vi "ParseSpec.vi"(8 "error in (no error)":errorcluster, 11 "Spec XML":string="<?xml version=\"1.0\" encoding=\"utf-8\"?>\n<Medulla>\n  <Doctype>Result</Doctype>\n  <Checksum>8765544332</Checksum>\n  <DriverKey>86y2e783he87</DriverKey>\n  <SpecId>1234567</SpecId>\n  <TransactionId>672362836</TransactionId>\n  <AccountID>Audinate</AccountID>\n  <SpecName>QF_TestSpec_CI24RE</SpecName>\n  <WorkflowStep>Test_CoilQF</WorkflowStep>\n  <SerialNumber>87362736</SerialNumber>\n  <BatchNumber>ase</BatchNumber>\n  <Status>Pass</Status>\n  <Comment>Repaired Unit</Comment>\n  <FirstFail>42344</FirstFail>\n  <Employee>Kurt</Employee>\n  <LocalMachine>QTS_Rig_1</LocalMachine>\n  <ResourceKey>12yu2yheiuh3</ResourceKey>\n  <Date>18/7/17</Date>\n  <Time>13:23:56</Time>\n  <Duration>00:1:27</Duration>\n  <DUTPosition>1</DUTPosition>\n  <Components>\n    <Component>\n      <SerialNumber>23214</SerialNumber>\n      <PartNumber>1234</PartNumber>\n      <Revision>A</Revision>\n      <BatchNumber></BatchNumber>\n      <Name>Grism</Name>\n      <Description>The Grism</Description>\n      <Attached>No</Attached>\n    </Component>\n    <Component>\n      <SerialNumber>464646646</SerialNumber>\n      <PartNumber>3456</PartNumber>\n      <Revision>B</Revision>\n      <BatchNumber></BatchNumber>\n      <Name>Prism</Name>\n      <Description>The Prism</Description>\n      <Attached>Yes</Attached>\n    </Component>\n  </Components>\n  <Attributes>\n    <Attribute>\n      <Name>Address</Name>\n      <Description>The IP of the Unit</Description>\n      <DataType>String</DataType>\n      <Value>192.168.1.7</Value>\n<DisplayFormat>%.3f</DisplayFormat>\n      <Access>R</Access>\n      <Required>NA</Required>\n    </Attribute>\n    <Attribute>\n      <Name>BaudRate</Name>\n      <Description>Baud rate of com port</Description>\n      <DataType>Int</DataType>\n      <Value>9600</Value>\n<DisplayFormat></DisplayFormat>\n      <Access>W</Access>\n      <Required>Yes</Required>\n    </Attribute>\n    <Attribute>\n      <Name>Switch State</Name>\n      <Description>State of the switch</Description>\n      <DataType>Boolean</DataType>\n      <Value>True</Value>\n<DisplayFormat></DisplayFormat>\n      <Access>W</Access>\n      <Required>No</Required>\n    </Attribute>\n  </Attributes>\n  <Tests>\n    <Test>\n      <Code>1</Code>\n      <Name>QFM Tests</Name>\n      <Description>blah</Description>\n      <Group></Group>\n      <IsGroup>Yes</IsGroup>\n      <Tag>QFM Tests</Tag>\n      <Method></Method>\n      <Parameter />\n      <DataType>Boolean</DataType>\n      <Value>1</Value>\n      <Status>Pass</Status>\n      <LimitLo></LimitLo>\n      <LimitHi></LimitHi>\n      <StringMatch></StringMatch>\n      <BooleanMatch>1</BooleanMatch>\n      <DisplayFormat></DisplayFormat>\n      <Units></Units>\n      <TestTime>00:01:27</TestTime>\n    </Test>\n    <Test>\n      <Code>1.1</Code>\n      <Name>Test Signal Strength</Name>\n      <Description>Test the signal strength</Description>\n      <Group>QFM Tests</Group>\n      <IsGroup>No</IsGroup>\n      <Tag>QFM Tests:Test Signal Strength</Tag>\n      <Method>Test_Sig</Method>\n      <Parameter />\n      <DataType>Int</DataType>\n      <Value>34.56</Value>\n      <Status>Pass</Status>\n      <LimitLo>25</LimitLo>\n      <LimitHi>100</LimitHi>\n      <StringMatch></StringMatch>\n      <BooleanMatch></BooleanMatch>\n      <DisplayFormat>%d</DisplayFormat>\n      <Units>Watts</Units>\n      <TestTime>00:00:45</TestTime>\n    </Test>\n    <Test>\n      <Code>1.2</Code>\n      <Name>Test Signal Frequency</Name>\n      <Description>Test the signal frequency</Description>\n      <Group>QFM Tests</Group>\n      <IsGroup>No</IsGroup>\n      <Tag>QFM Tests:Test Signal Frequency</Tag>\n      <Method>Test_Freq</Method>\n      <Parameter />\n      <DataType>Dbl</DataType>\n      <Value>45.67</Value>\n      <Status>Pass</Status>\n      <LimitLo>45</LimitLo>\n      <LimitHi>46</LimitHi>\n      <StringMatch></StringMatch>\n      <BooleanMatch></BooleanMatch>\n      <DisplayFormat>%.3f</DisplayFormat>\n      <Units>MHz</Units>\n      <TestTime>00:00:20</TestTime>\n    </Test>\n    <Test>\n      <Code>Code</Code>\n      <Name>Test Firmware Vesion</Name>\n      <Description>Test the Firmware Vesion</Description>\n      <Group>QFM Tests</Group>\n      <IsGroup>No</IsGroup>\n      <Tag>QFM Tests:Test Firmware Vesion</Tag>\n      <Method>Test_FWVer</Method>\n      <Parameter />\n      <DataType>String</DataType>\n      <Value>Ver1.2</Value>\n      <Status>Pass</Status>\n      <LimitLo></LimitLo>\n      <LimitHi></LimitHi>\n      <StringMatch>Ver1.2</StringMatch>\n      <BooleanMatch></BooleanMatch>\n      <DisplayFormat></DisplayFormat>\n      <Units></Units>\n      <TestTime>00:00:12</TestTime>\n    </Test>\n    <Test>\n      <Code>Test LED State</Code>\n      <Name>Test LED State</Name>\n      <Description>Tests that the LED is On</Description>\n      <Group>QFM Tests</Group>\n      <IsGroup>No</IsGroup>\n      <Tag>QFM Tests:Test LED State</Tag>\n      <Method>Test_LED</Method>\n      <Parameter />\n      <DataType>Boolean</DataType>\n      <Value>True</Value>\n      <Status>Pass</Status>\n      <LimitLo></LimitLo>\n      <LimitHi></LimitHi>\n      <StringMatch></StringMatch>\n      <BooleanMatch>True</BooleanMatch>\n      <DisplayFormat></DisplayFormat>\n      <Units></Units>\n      <TestTime>00:00:10</TestTime>\n    </Test>\n  </Tests>\n</Medulla>") -> (0 "error out":errorcluster, 3 "Spec":T1)   [LabVIEW 2022 SP3, in "MES_Base.lvlib" / "MES_Base.lvclass"]
uses:
  MES_Base.lvclass
  Controls/Spec.ctl
  Controls/SpecHeader.ctl
  Controls/Status.ctl
  Controls/SpecComponent.ctl
  Controls/SpecAttribute.ctl
  Controls/DataType.ctl
  Controls/Test.ctl
  <vilib>/xml/Load XML String.vi
  <vilib>/xml/Close Reference(Node).vi
  <vilib>/xml/NI_XML.lvlib
panel:
  # "<SerialNumber>23214</SerialNumber>\n      <PartNumber>1234</PartNumber>\n      <Revision>A</Revision>\n      <BatchNumber></BatchNumber>\n      <Name>Grism</Name>\n      <Description>The Grism</Description>\n      <Attached>Yes</Attached>"
  # "<Attribute>\n      <Name>Address</Name>\n      <Description>The IP of the Unit</Description>\n      <DataType>String</DataType>\n      <Value>192.168.1.7</Value>\n      <Access>R</Access>\n      <Required>NA</Required>\n    </Attribute>"
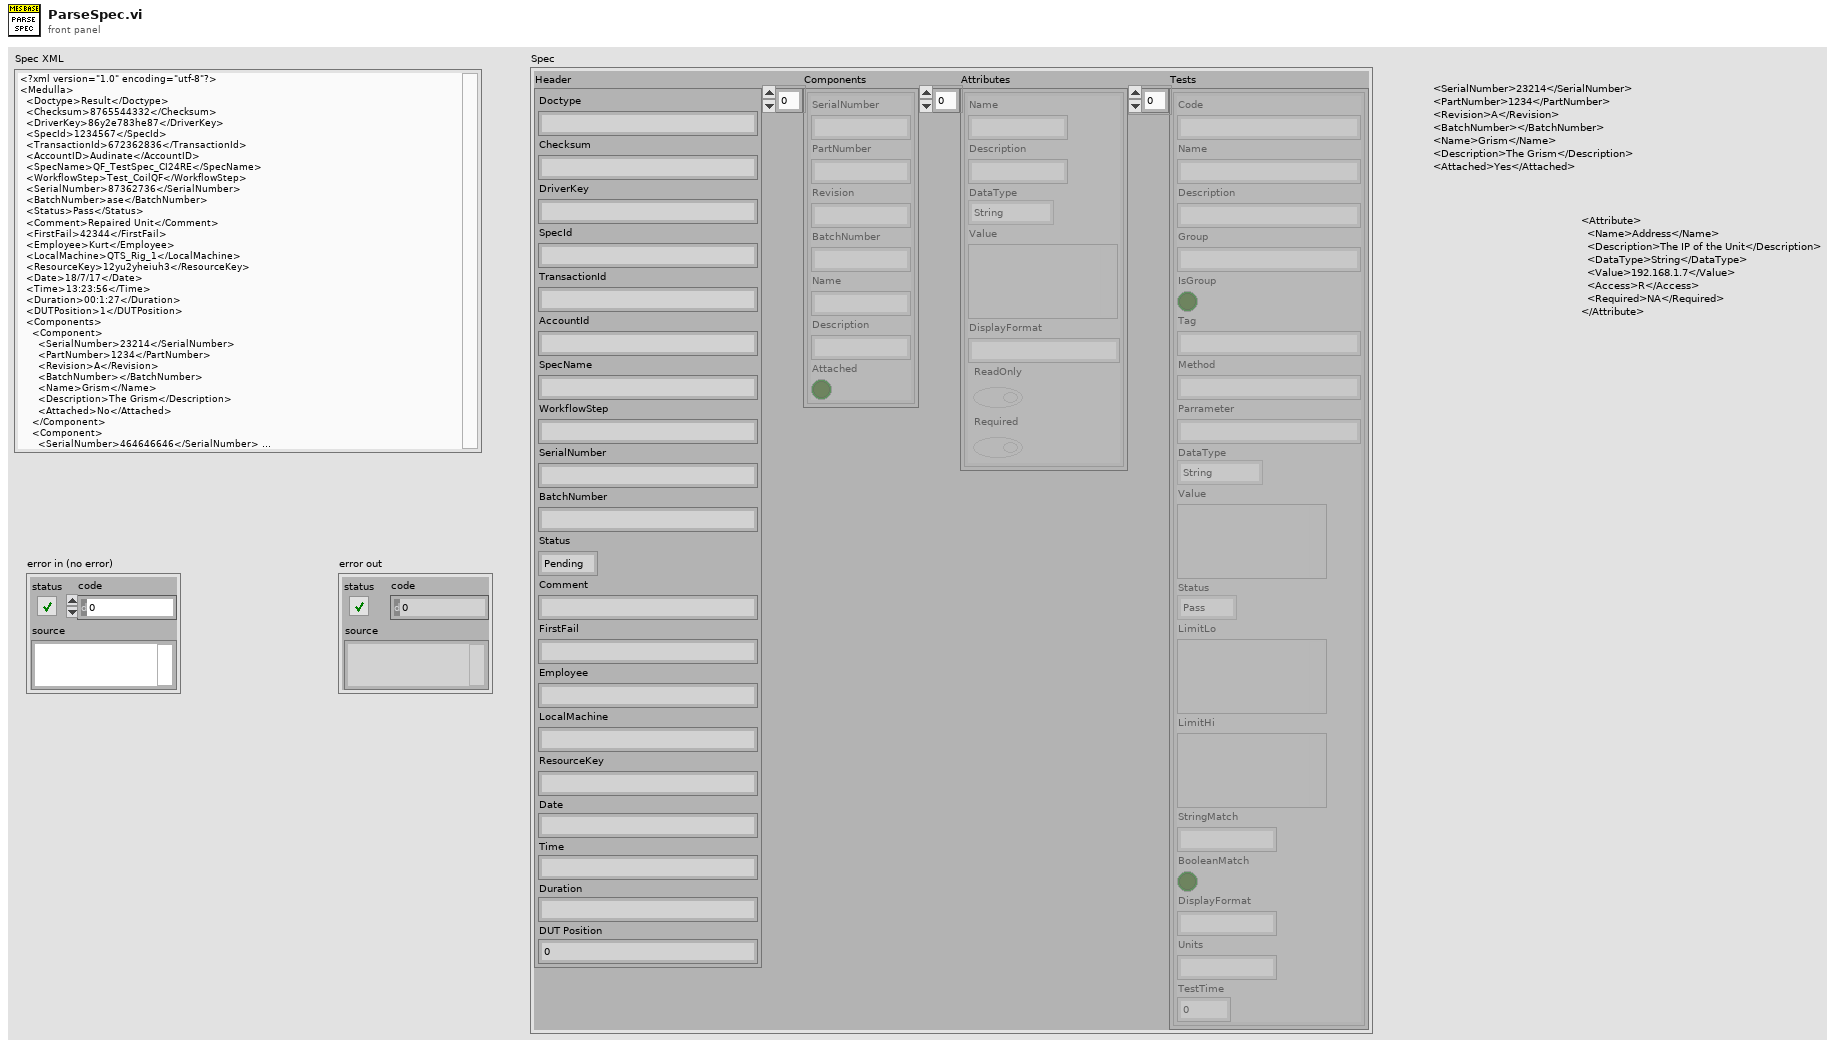
[diagram p1: front panel]
types:
  T1 = typedef "MES_Base.lvlib/MES_Base.lvclass/Spec.ctl" = cluster{"Header":T2, "Components":T4[], "Attributes":T5[], "Tests":T7[]}
  T2 = typedef "MES_Base.lvlib/MES_Base.lvclass/SpecHeader.ctl" = cluster{"Doctype":string, "Checksum":string, "DriverKey":string, "SpecId":string, "TransactionId":string, "AccountId":string, "SpecName":string, "WorkflowStep":string, "SerialNumber":string, "BatchNumber":string, "Status":T3, "Comment":string, "FirstFail":string, "Employee":string, "LocalMachine":string, "ResourceKey":string, "Date":string, "Time":string, "Duration":string, "DUT Position":i32}
  T3 = typedef "MES_Base.lvlib/MES_Base.lvclass/Status.ctl" = enum16{"Pending", "Pass", "Fail"}
  T4 = typedef "MES_Base.lvlib/MES_Base.lvclass/SpecComponent.ctl" = cluster{"SerialNumber":string, "PartNumber":string, "Revision":string, "BatchNumber":string, "Name":string, "Description":string, "Attached":bool}
  T5 = typedef "MES_Base.lvlib/MES_Base.lvclass/SpecAttribute.ctl" = cluster{"Name":string, "Description":string, "DataType":T6, "Value":variant, "DisplayFormat":string, "ReadOnly":bool, "Required":bool}
  T6 = typedef "MES_Base.lvlib/MES_Base.lvclass/DataType.ctl" = enum16{"NA", "String", "Boolean", "Int", "Dbl"}
  T7 = typedef "MES_Base.lvlib/MES_Base.lvclass/Test.ctl" = cluster{"Code":string, "Name":string, "Description":string, "Group":string, "IsGroup":bool, "Tag":string, "Method":string, "Parrameter":string, "DataType":T6, "Value":variant, "Status":T3, "LimitLo":variant, "LimitHi":variant, "StringMatch":string, "BooleanMatch":bool, "DisplayFormat":string, "Units":string, "TestTime":dbl}
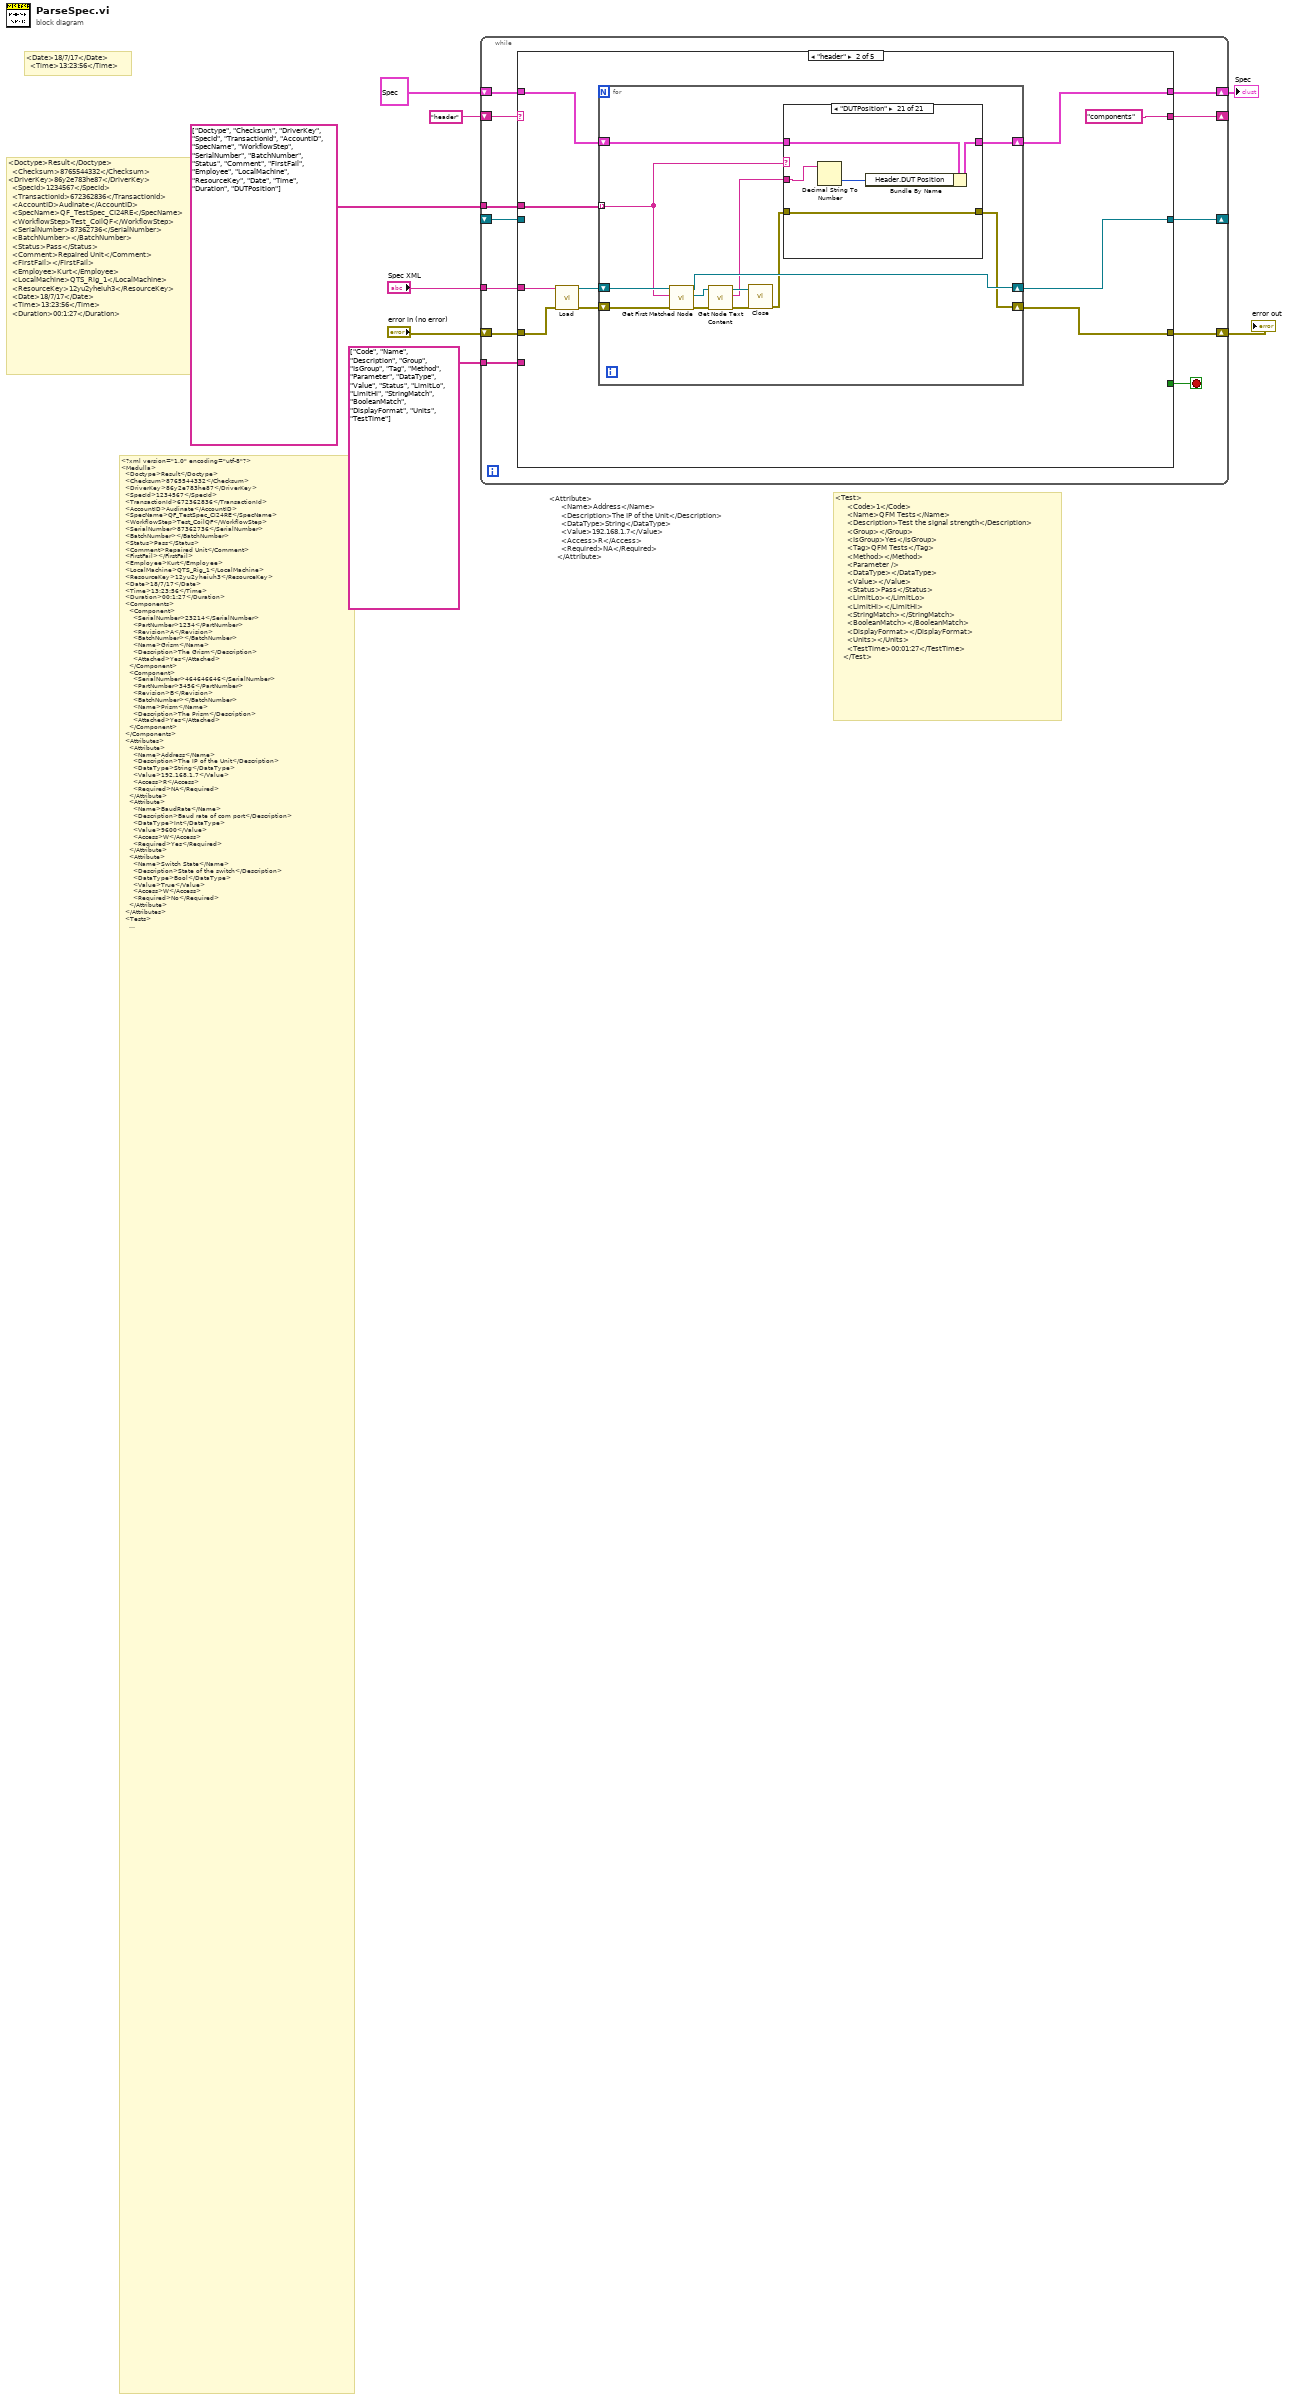
[diagram p0: block diagram]
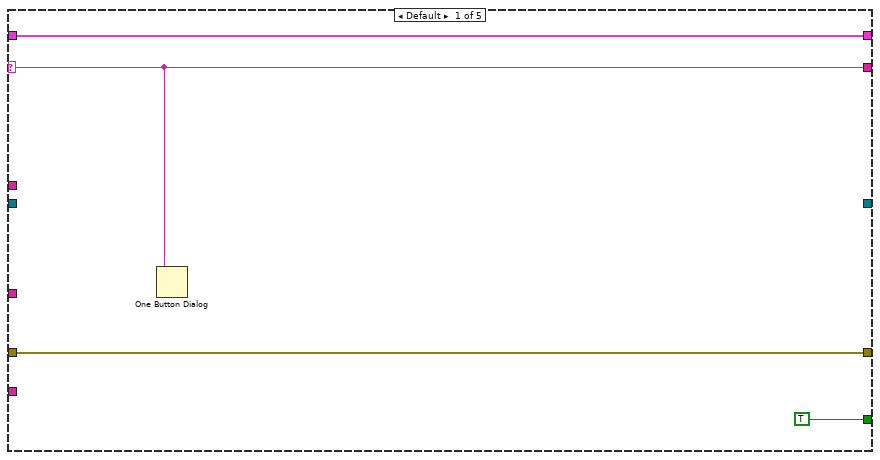
[diagram p2: hidden frame]
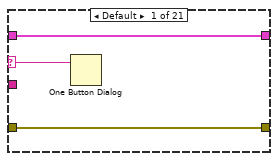
[diagram p3: hidden frame]
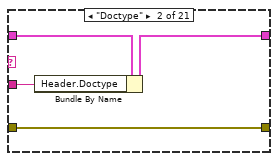
[diagram p4: hidden frame]
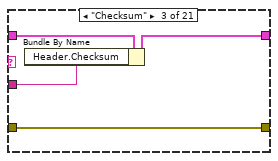
[diagram p5: hidden frame]
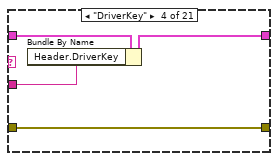
[diagram p6: hidden frame]
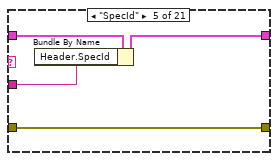
[diagram p7: hidden frame]
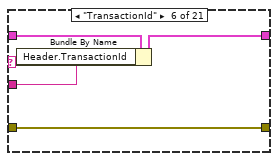
[diagram p8: hidden frame]
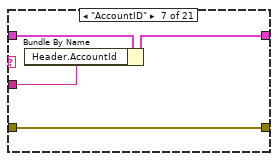
[diagram p9: hidden frame]
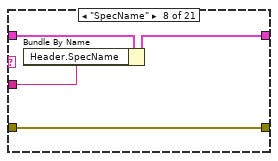
[diagram p10: hidden frame]
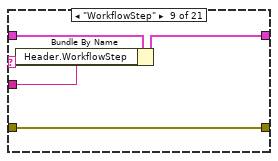
[diagram p11: hidden frame]
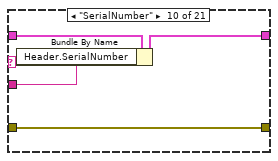
[diagram p12: hidden frame]
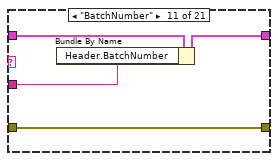
[diagram p13: hidden frame]
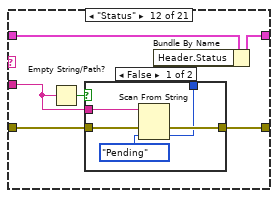
[diagram p14: hidden frame]
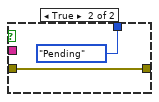
[diagram p15: hidden frame]
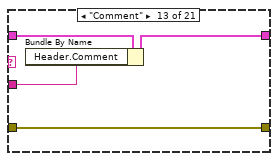
[diagram p16: hidden frame]
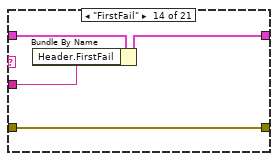
[diagram p17: hidden frame]
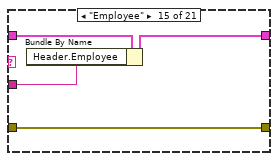
[diagram p18: hidden frame]
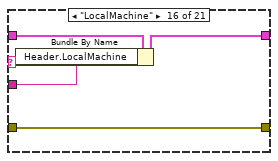
[diagram p19: hidden frame]
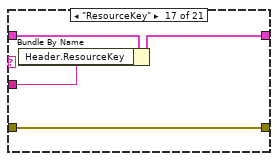
[diagram p20: hidden frame]
diagram:
  # "<Date>18/7/17</Date>\n  <Time>13:23:56</Time>"
  # "<Test>\n      <Code>1</Code>\n      <Name>QFM Tests</Name>\n      <Description>Test the signal strength</Description>\n      <Group></Group>\n      <IsGroup>Yes</IsGroup>\n      <Tag>QFM Tests</Tag>\n      <Method></Method>\n      <Parameter />\n      <DataType></DataType>\n      <Value></Value>\n      <Status>Pass</Status>\n      <LimitLo></LimitLo>\n      <LimitHi></LimitHi>\n      <StringMatch></StringMatch>\n      <BooleanMatch></BooleanMatch>\n      <DisplayFormat></DisplayFormat>\n      <Units></Units>\n      <TestTime>00:01:27</TestTime>\n    </Test>"
  # "<Attribute>\n      <Name>Address</Name>\n      <Description>The IP of the Unit</Description>\n      <DataType>String</DataType>\n      <Value>192.168.1.7</Value>\n      <Access>R</Access>\n      <Required>NA</Required>\n    </Attribute>"
  # "<Doctype>Result</Doctype>\n  <Checksum>8765544332</Checksum>\n<DriverKey>86y2e783he87</DriverKey>\n  <SpecId>1234567</SpecId>\n  <TransactionId>672362836</TransactionId>\n  <AccountID>Audinate</AccountID>\n  <SpecName>QF_TestSpec_CI24RE</SpecName>\n  <WorkflowStep>Test_CoilQF</WorkflowStep>\n  <SerialNumber>87362736</SerialNumber>\n  <BatchNumber></BatchNumber>\n  <Status>Pass</Status>\n  <Comment>Repaired Unit</Comment>\n  <FirstFail></FirstFail>\n  <Employee>Kurt</Employee>\n  <LocalMachine>QTS_Rig_1</LocalMachine>\n  <ResourceKey>12yu2yheiuh3</ResourceKey>\n  <Date>18/7/17</Date>\n  <Time>13:23:56</Time>\n  <Duration>00:1:27</Duration>"
  # "<?xml version=\"1.0\" encoding=\"utf-8\"?>\n<Medulla>\n  <Doctype>Result</Doctype>\n  <Checksum>8765544332</Checksum>\n  <DriverKey>86y2e783he87</DriverKey>\n  <SpecId>1234567</SpecId>\n  <TransactionId>672362836</TransactionId>\n  <AccountID>Audinate</AccountID>\n  <SpecName>QF_TestSpec_CI24RE</SpecName>\n  <WorkflowStep>Test_CoilQF</WorkflowStep>\n  <SerialNumber>87362736</SerialNumber>\n  <BatchNumber></BatchNumber>\n  <Status>Pass</Status>\n  <Comment>Repaired Unit</Comment>\n  <FirstFail></FirstFail>\n  <Employee>Kurt</Employee>\n  <LocalMachine>QTS_Rig_1</LocalMachine>\n  <ResourceKey>12yu2yheiuh3</ResourceKey>\n  <Date>18/7/17</Date>\n  <Time>13:23:56</Time>\n  <Duration>00:1:27</Duration>\n  <Components>\n    <Component>\n      <SerialNumber>23214</SerialNumber>\n      <PartNumber>1234</PartNumber>\n      <Revision>A</Revision>\n      <BatchNumber></BatchNumber>\n      <Name>Grism</Name>\n      <Description>The Grism</Description>\n      <Attached>Yes</Attached>\n    </Component>\n    <Component>\n      <SerialNumber>464646646</SerialNumber>\n      <PartNumber>3456</PartNumber>\n      <Revision>B</Revision>\n      <BatchNumber></BatchNumber>\n      <Name>Prism</Name>\n      <Description>The Prism</Description>\n      <Attached>Yes</Attached>\n    </Component>\n  </Components>\n  <Attributes>\n    <Attribute>\n      <Name>Address</Name>\n      <Description>The IP of the Unit</Description>\n      <DataType>String</DataType>\n      <Value>192.168.1.7</Value>\n      <Access>R</Access>\n      <Required>NA</Required>\n    </Attribute>\n    <Attribute>\n      <Name>BaudRate</Name>\n      <Description>Baud rate of com port</Description>\n      <DataType>Int</DataType>\n      <Value>9600</Value>\n      <Access>W</Access>\n      <Required>Yes</Required>\n    </Attribute>\n    <Attribute>\n      <Name>Switch State</Name>\n      <Description>State of the switch</Description>\n      <DataType>Bool</DataType>\n      <Value>True</Value>\n      <Access>W</Access>\n      <Required>No</Required>\n    </Attribute>\n  </Attributes>\n  <Tests>\n    <Test>\n      <Code>1</Code>\n      <Name>QFM Tests</Name>\n      <Description>Test the signal strength</Description>\n      <Group></Group>\n      <IsGroup>Yes</IsGroup>\n      <Tag>QFM Tests</Tag>\n      <Method></Method>\n      <Parameter />\n      <DataType></DataType>\n      <Value></Value>\n      <Status>Pass</Status>\n      <LimitLo></LimitLo>\n      <LimitHi></LimitHi>\n      <StringMatch></StringMatch>\n      <BooleanMatch></BooleanMatch>\n      <DisplayFormat></DisplayFormat>\n      <Units></Units>\n      <TestTime>00:01:27</TestTime>\n    </Test>\n    <Test>\n      <Code>1.1</Code>\n      <Name>Test Signal Strength</Name>\n      <Description>Test the signal strength</Description>\n      <Group>QFM Tests</Group>\n      <IsGroup>No</IsGroup>\n      <Tag>QFM Tests:Test Signal Strength</Tag>\n      <Method>Test_Sig</Method>\n      <Parameter />\n      <DataType>Int</DataType>\n      <Value>34.56</Value>\n      <Status>Pass</Status>\n      <LimitLo>25</LimitLo>\n      <LimitHi>100</LimitHi>\n      <StringMatch></StringMatch>\n      <BooleanMatch></BooleanMatch>\n      <DisplayFormat>%d</DisplayFormat>\n      <Units>Watts</Units>\n      <TestTime>00:00:45</TestTime>\n    </Test>\n    <Test>\n      <Code>1.2</Code>\n      <Name>Test Signal Frequency</Name>\n      <Description>Test the signal frequency</Description>\n      <Group>QFM Tests</Group>\n      <IsGroup>No</IsGroup>\n      <Tag>QFM Tests:Test Signal Frequency</Tag>\n      <Method>Test_Freq</Method>\n      <Parameter />\n      <DataType>DBL</DataType>\n      <Value>45.67</Value>\n      <Status>Pass</Status>\n      <LimitLo>45</LimitLo>\n      <LimitHi>46</LimitHi>\n      <StringMatch></StringMatch>\n      <BooleanMatch></BooleanMatch>\n      <DisplayFormat>%.3f</DisplayFormat>\n      <Units>MHz</Units>\n      <TestTime>00:00:20</TestTime>\n    </Test>\n    <Test>\n      <Code>Code</Code>\n      <Name>Test Firmware Vesion</Name>\n      <Description>Test the Firmware Vesion</Description>\n      <Group>QFM Tests</Group>\n      <IsGroup>No</IsGroup>\n      <Tag>QFM Tests:Test Firmware Vesion</Tag>\n      <Method>Test_FWVer</Method>\n      <Parameter />\n      <DataType>String</DataType>\n      <Value>Ver1.2</Value>\n      <Status>Pass</Status>\n      <LimitLo></LimitLo>\n      <LimitHi></LimitHi>\n      <StringMatch>Ver1.2</StringMatch>\n      <BooleanMatch></BooleanMatch>\n      <DisplayFormat></DisplayFormat>\n      <Units></Units>\n      <TestTime>00:00:12</TestTime>\n    </Test>\n    <Test>\n      <Code>Test LED State</Code>\n      <Name>Test LED State</Name>\n      <Description>Tests that the LED is On</Description>\n      <Group>QFM Tests</Group>\n      <IsGroup>No</IsGroup>\n      <Tag>QFM Tests:Test LED State</Tag>\n      <Method>Test_LED</Method>\n      <Parameter />\n      <DataType>Boolean</DataType>\n      <Value>True</Value>\n      <Status>True</Status>\n      <LimitLo></LimitLo>\n      <LimitHi></LimitHi>\n      <StringMatch></StringMatch>\n      <BooleanMatch>True</BooleanMatch>\n      <DisplayFormat></DisplayFormat>\n      <Units></Units>\n      <TestTime>00:00:10</TestTime>\n    </Test>\n  </Tests>\n</Medulla>"
  n1 = while {
    shift-right: [w15] -> w4
    shift-left: "error in (no error)" -> [w19]
    tunnel: "Spec XML" -> [w18]
    shift-right: [w13] -> _
    shift-left: "header" -> [w20]
    shift-right: [w14] -> w2
    shift-left: T1 {"Header"={"Doctype"="", "Checksum"="", "DriverKey"="", "SpecId"="", "TransactionId"="", "AccountId"="", "SpecName"="", "WorkflowStep"="", "SerialNumber"="", "BatchNumber"="", "Status"=enum."Pending", "Comment"="", "FirstFail"="", "Employee"="", "LocalMachine"="", "ResourceKey"="", "Date"="", "Time"="", "Duration"="", "DUT Position"=0}, "Components"=[], "Attributes"=[], "Tests"=[]} ("Spec") -> [w17]
    tunnel: string[] ["Doctype", "Checksum", "DriverKey", "SpecId", "TransactionId", "AccountID", "SpecName", "WorkflowStep", "SerialNumber", "BatchNumber", "Status", "Comment", "FirstFail", "Employee", "LocalMachine", "ResourceKey", "Date", "Time", "Duration", "DUTPosition"] -> [w16]
    shift-right: [w11] -> _
    shift-left: _ -> [w10]
    tunnel: string[] ["Code", "Name", "Description", "Group", "IsGroup", "Tag", "Method", "Parameter", "DataType", "Value", "Status", "LimitLo", "LimitHi", "StringMatch", "BooleanMatch", "DisplayFormat", "Units", "TestTime"] -> [w9]
    stop <- w12 stop-if-true
    n2 = case shown="\"header\"" w20 {
      selector: w20 -> [w21 _ _ _ _]
      tunnel: w19 -> [w24 w33 w152 w204 w286]
      tunnel: w18 -> [_ w34 _ _ _]
      tunnel: w17 -> [w22 w29 w146 w198 w281]
      tunnel: w16 -> [_ w30 _ _ _]
      tunnel: [w24 w28 w148 w200 w282] -> w15
      tunnel: [w22 w27 w145 w197 w280] -> w14
      tunnel: [w21 "components" "attributes" "tests" "done"] -> w13
      tunnel: [TRUE _ _ _ TRUE] -> w12
      tunnel: [_ w25 w143 w195 w278] -> w11
      tunnel: w10 -> [_ _ w143 w195 w278]
      tunnel: w9 -> [_ _ _ _ w276]
      frame Default {
        n3 = One Button Dialog(message=w21) -> ()  [unwired: 1 in, 1 out]
      }
      frame "header" {
        n4 = call-poly <vilib>:"Load.vi"("XML string"=w34, "error in (no error)"=w33) -> ("DOM document out"=w32:refnum<k20>, "error out"=w31:errorcluster)  [unwired: 11 in, 1 out]
        n5 = for {
          shift-right: [w35] -> w28
          shift-left: w31 -> [w38]
          tunnel: w30 -> [w37] mode=indexing
          shift-right: [w42] -> w25
          shift-left: w32 -> [w47]
          shift-right: [w39] -> w27
          shift-left: w29 -> [w41]
          n6 = call <vilib>:"Get First Matched Node.vi"("error in (no error)"=w38, "XPath expression"=w37, "node in"=w47) -> ("error out"=w46:errorcluster, "node result"=w45:refnum<k20>, "node out"=w42:refnum<k20>)  [unwired: 6 in]
          n7 = call <vilib>:"Get Node Text Content.vi"("error in (no error)"=w46, "node in"=w45) -> ("error out"=w44:errorcluster, "node text"=w40:string, "node out"=w43:refnum<k20>)  [unwired: 7 in]
          n8 = call-poly <vilib>:"Close.vi"("error in (no error)"=w44, "node"=w43) -> ("error out"=w36:errorcluster)  [unwired: 7 out]
          n9 = case shown="\"DUTPosition\"" w37 {
            selector: w37 -> [w49 _ _ _ _ _ _ _ _ _ _ _ _ _ _ _ _ _ _ _ _]
            tunnel: w41 -> [w50 w54 w58 w62 w66 w70 w74 w78 w82 w86 w90 w97 w108 w112 w116 w120 w124 w128 w132 w136 w141]
            tunnel: w40 -> [_ w52 w56 w60 w64 w68 w72 w76 w80 w84 w88 w93 w106 w110 w114 w118 w122 w126 w130 w134 w138]
            tunnel: [w50 w53 w57 w61 w65 w69 w73 w77 w81 w85 w89 w96 w107 w111 w115 w119 w123 w127 w131 w135 w140] -> w39
            tunnel: w36 -> [w48 w51 w55 w59 w63 w67 w71 w75 w79 w83 w87 w92 w105 w109 w113 w117 w121 w125 w129 w133 w139]
            tunnel: [w48 w51 w55 w59 w63 w67 w71 w75 w79 w83 w87 w91 w105 w109 w113 w117 w121 w125 w129 w133 w139] -> w35
            frame Default {
              n10 = One Button Dialog(message=w49) -> ()  [unwired: 1 in, 1 out]
            }
            frame "Doctype" {
              n11 = Bundle By Name(cluster=w54, "Header.Doctype"=w52) -> (w53:T1)
            }
            frame "Checksum" {
              n12 = Bundle By Name(cluster=w58, "Header.Checksum"=w56) -> (w57:T1)
            }
            frame "DriverKey" {
              n13 = Bundle By Name(cluster=w62, "Header.DriverKey"=w60) -> (w61:T1)
            }
            frame "SpecId" {
              n14 = Bundle By Name(cluster=w66, "Header.SpecId"=w64) -> (w65:T1)
            }
            frame "TransactionId" {
              n15 = Bundle By Name(cluster=w70, "Header.TransactionId"=w68) -> (w69:T1)
            }
            frame "AccountID" {
              n16 = Bundle By Name(cluster=w74, "Header.AccountId"=w72) -> (w73:T1)
            }
            frame "SpecName" {
              n17 = Bundle By Name(cluster=w78, "Header.SpecName"=w76) -> (w77:T1)
            }
            frame "WorkflowStep" {
              n18 = Bundle By Name(cluster=w82, "Header.WorkflowStep"=w80) -> (w81:T1)
            }
            frame "SerialNumber" {
              n19 = Bundle By Name(cluster=w86, "Header.SerialNumber"=w84) -> (w85:T1)
            }
            frame "BatchNumber" {
              n20 = Bundle By Name(cluster=w90, "Header.BatchNumber"=w88) -> (w89:T1)
            }
            frame "Status" {
              n21 = Empty String/Path?(string/path=w93) -> (empty?=w95:bool)
              n22 = case shown="False" w95 {
                tunnel: w92 -> [w102 w104]
                tunnel: [w101 w104] -> w91
                tunnel: [w99 Status."Pending" ("Status")] -> w94
                tunnel: w93 -> [w98 _]
                frame False {
                  n23 = Scan From String(input string=w98, error in=w102, default 1=Status."Pending" ("Status")) -> (error out=w101:errorcluster, output 1=w99:T3)  [unwired: 2 in, 2 out]
                }
                frame True {
                }
              }
              n24 = Bundle By Name(cluster=w97, "Header.Status"=w94) -> (w96:T1)
            }
            frame "Comment" {
              n25 = Bundle By Name(cluster=w108, "Header.Comment"=w106) -> (w107:T1)
            }
            frame "FirstFail" {
              n26 = Bundle By Name(cluster=w112, "Header.FirstFail"=w110) -> (w111:T1)
            }
            frame "Employee" {
              n27 = Bundle By Name(cluster=w116, "Header.Employee"=w114) -> (w115:T1)
            }
            frame "LocalMachine" {
              n28 = Bundle By Name(cluster=w120, "Header.LocalMachine"=w118) -> (w119:T1)
            }
            frame "ResourceKey" {
              n29 = Bundle By Name(cluster=w124, "Header.ResourceKey"=w122) -> (w123:T1)
            }
            frame "Date" {
              n30 = Bundle By Name(cluster=w128, "Header.Date"=w126) -> (w127:T1)
            }
            frame "Time" {
              n31 = Bundle By Name(cluster=w132, "Header.Time"=w130) -> (w131:T1)
            }
            frame "Duration" {
              n32 = Bundle By Name(cluster=w136, "Header.Duration"=w134) -> (w135:T1)
            }
            frame "DUTPosition" {
              n33 = Decimal String To Number(string=w138) -> (number=w137:i32)  [unwired: 2 in, 1 out]
              n34 = Bundle By Name(cluster=w141, "Header.DUT Position"=w137) -> (w140:T1)
            }
          }
        }
      }
      frame "components" {
        n35 = call <vilib>:"Get All Matched Nodes.vi"("error in (no error)"=w152, "XPath expression"="Components/Component", "node in"=w143) -> ("error out"=w150:errorcluster, "node result array"=w149:refnum<k20>[])  [unwired: 6 in, 1 out]
        n36 = for {
          shift-right: [w155] -> w148
          shift-left: w150 -> [w158]
          tunnel: w149 -> [w157] mode=indexing
          tunnel: string[] ["SerialNumber", "PartNumber", "Revision", "BatchNumber", "Name", "Description", "Attached"] -> [w156]
          tunnel: [w154] -> w144 mode=indexing
          n37 = for {
            tunnel: w157 -> [w168]
            tunnel: w156 -> [w162] mode=indexing
            shift-right: [w164] -> w155
            shift-left: w158 -> [w169]
            shift-right: [w160] -> w154
            shift-left: T4 {"SerialNumber"="", "PartNumber"="", "Revision"="", "BatchNumber"="", "Name"="", "Description"="", "Attached"=FALSE} ("Component") -> [w161]
            n38 = call <vilib>:"Get First Matched Node.vi"("error in (no error)"=w169, "XPath expression"=w162, "node in"=w168) -> ("error out"=w166:errorcluster, "node result"=w167:refnum<k20>)  [unwired: 6 in, 1 out]
            n39 = call <vilib>:"Get Node Text Content.vi"("error in (no error)"=w166, "node in"=w167) -> ("error out"=w165:errorcluster, "node text"=w159:string, "node out"=w163:refnum<k20>)  [unwired: 7 in]
            n40 = case shown="\"Revision\"" w162 {
              tunnel: w161 -> [w170 w173 w176 w179 w182 w185 w188 w193]
              tunnel: [w170 w172 w175 w178 w181 w184 w187 w192] -> w160
              tunnel: w159 -> [_ w171 w174 w177 w180 w183 w186 w191]
              frame Default {
              }
              frame "SerialNumber" {
                n41 = Bundle By Name(cluster=w173, "SerialNumber"=w171) -> (w172:T4)
              }
              frame "PartNumber" {
                n42 = Bundle By Name(cluster=w176, "PartNumber"=w174) -> (w175:T4)
              }
              frame "Revision" {
                n43 = Bundle By Name(cluster=w179, "Revision"=w177) -> (w178:T4)
              }
              frame "BatchNumber" {
                n44 = Bundle By Name(cluster=w182, "BatchNumber"=w180) -> (w181:T4)
              }
              frame "Name" {
                n45 = Bundle By Name(cluster=w185, "Name"=w183) -> (w184:T4)
              }
              frame "Description" {
                n46 = Bundle By Name(cluster=w188, "Description"=w186) -> (w187:T4)
              }
              frame "Attached" {
                n47 = Equal?(x="Yes", y=w191) -> (x = y?=w189:bool)
                n48 = Bundle By Name(cluster=w193, "Attached"=w189) -> (w192:T4)
              }
            }
            n49 = call-poly <vilib>:"Close.vi"("error in (no error)"=w165, "node"=w163) -> ("error out"=w164:errorcluster)  [unwired: 7 in]
          }
        }
        n50 = Bundle By Name(cluster=w146, "Components"=w144) -> (w145:T1)
      }
      frame "attributes" {
        n51 = call <vilib>:"Get All Matched Nodes.vi"("error in (no error)"=w204, "XPath expression"="Attributes/Attribute", "node in"=w195) -> ("error out"=w202:errorcluster, "node result array"=w201:refnum<k20>[])  [unwired: 6 in, 1 out]
        n52 = for {
          shift-right: [w207] -> w200
          shift-left: w202 -> [w210]
          tunnel: w201 -> [w209] mode=indexing
          tunnel: string[] ["Name", "Description", "DataType", "Value", "DisplayFormat", "Access", "Required"] -> [w208]
          tunnel: [w206] -> w196 mode=indexing
          n53 = for {
            tunnel: w209 -> [w221]
            tunnel: w208 -> [w216] mode=indexing
            shift-right: [w218] -> w207
            shift-left: w210 -> [w222]
            shift-right: [w214] -> w206
            shift-left: T5 {"Name"="", "Description"="", "DataType"=enum."String", "Value"=variant, "DisplayFormat"="", "ReadOnly"=FALSE, "Required"=FALSE} ("Attribute") -> [w215]
            n54 = call <vilib>:"Get First Matched Node.vi"("error in (no error)"=w222, "XPath expression"=w216, "node in"=w221) -> ("error out"=w219:errorcluster, "node result"=w220:refnum<k20>)  [unwired: 6 in, 1 out]
            n55 = call <vilib>:"Get Node Text Content.vi"("error in (no error)"=w219, "node in"=w220) -> ("error out"=w212:errorcluster, "node text"=w213:string, "node out"=w217:refnum<k20>)  [unwired: 7 in]
            n56 = case shown="\"DataType\"" w216 {
              tunnel: w215 -> [w224 w228 w232 w239 w243 w260 w268 w274]
              tunnel: [w224 w227 w231 w238 w245 w262 w267 w273] -> w214
              tunnel: w213 -> [_ w226 w230 w237 w241 w259 w266 w271]
              tunnel: w212 -> [w223 w225 w229 w235 w244 w261 w263 w269]
              tunnel: [w223 w225 w229 w234 w244 w261 w263 w269] -> w211
              frame Default {
              }
              frame "Name" {
                n57 = Bundle By Name(cluster=w228, "Name"=w226) -> (w227:T5)
              }
              frame "Description" {
                n58 = Bundle By Name(cluster=w232, "Description"=w230) -> (w231:T5)
              }
              frame "DataType" {
                n59 = Scan From String(input string=w237, error in=w235, default 1=DataType."Dbl" ("DataType")) -> (error out=w234:errorcluster, output 1=w236:T6)  [unwired: 2 in, 2 out]
                n60 = Bundle By Name(cluster=w239, "DataType"=w236) -> (w238:T5)
              }
              frame "Value" {
                n61 = Unbundle By Name(w243) -> ("DataType"=w242:T6)
                n62 = case shown="\"Dbl\"" w242 {
                  tunnel: w241 -> [w247 w251 w255 w257]
                  tunnel: [w246 w248 w252 w258] -> w240
                  frame "String", Default {
                    n63 = To Variant(anything=w247) -> (Variant=w246:variant)
                  }
                  frame "Boolean" {
                    n64 = Equal?(x="1", y=w251) -> (x = y?=w249:bool)
                    n65 = To Variant(anything=w249) -> (Variant=w248:variant)
                  }
                  frame "Int" {
                    n66 = Decimal String To Number(string=w255, default (0L)=i64 0 ("default (0 I32)")) -> (number=w253:i64)  [unwired: 1 in, 1 out]
                    n67 = To Variant(anything=w253) -> (Variant=w252:variant)
                  }
                  frame "Dbl" {
                    n68 = Fract/Exp String To Number(string=w257) -> (number=w256:dbl)  [unwired: 3 in, 1 out]
                    n69 = To Variant(anything=w256) -> (Variant=w258:variant)
                  }
                }
                n70 = Bundle By Name(cluster=w243, "Value"=w240) -> (w245:T5)
              }
              frame "DisplayFormat" {
                n71 = Bundle By Name(cluster=w260, "DisplayFormat"=w259) -> (w262:T5)
              }
              frame "Access" {
                n72 = Equal?(x=w266, y="R") -> (x = y?=w264:bool)
                n73 = Bundle By Name(cluster=w268, "ReadOnly"=w264) -> (w267:T5)
              }
              frame "Required" {
                n74 = Equal?(x="Yes", y=w271) -> (x = y?=w270:bool)
                n75 = Bundle By Name(cluster=w274, "Required"=w270) -> (w273:T5)
              }
            }
            n76 = call-poly <vilib>:"Close.vi"("error in (no error)"=w211, "node"=w217) -> ("error out"=w218:errorcluster)  [unwired: 7 in]
          }
        }
        n77 = Bundle By Name(cluster=w198, "Attributes"=w196) -> (w197:T1)
      }
      frame "tests" {
        n78 = call <vilib>:"Get All Matched Nodes.vi"("error in (no error)"=w286, "XPath expression"="Tests/Test", "node in"=w278) -> ("error out"=w284:errorcluster, "node result array"=w283:refnum<k20>[])  [unwired: 6 in, 1 out]
        n79 = for {
          shift-right: [w289] -> w282
          shift-left: w284 -> [w292]
          tunnel: w283 -> [w291] mode=indexing
          tunnel: w276 -> [w290]
          tunnel: [w288] -> w279 mode=indexing
          n80 = for {
            tunnel: w291 -> [w303]
            tunnel: w290 -> [w298] mode=indexing
            shift-right: [w300] -> w289
            shift-left: w292 -> [w304]
            shift-right: [w296] -> w288
            shift-left: T7 {"Code"="", "Name"="", "Description"="", "Group"="", "IsGroup"=FALSE, "Tag"="", "Method"="", "Parrameter"="", "DataType"=enum."String", "Value"=variant, "Status"=enum."Pass", "LimitLo"=variant, "LimitHi"=variant, "StringMatch"="", "BooleanMatch"=FALSE, "DisplayFormat"="", "Units"="", "TestTime"=0.0} ("Cluster 2") -> [w297]
            n81 = call <vilib>:"Get First Matched Node.vi"("error in (no error)"=w304, "XPath expression"=w298, "node in"=w303) -> ("error out"=w301:errorcluster, "node result"=w302:refnum<k20>)  [unwired: 6 in, 1 out]
            n82 = call <vilib>:"Get Node Text Content.vi"("error in (no error)"=w301, "node in"=w302) -> ("error out"=w294:errorcluster, "node text"=w295:string, "node out"=w299:refnum<k20>)  [unwired: 7 in]
            n83 = case shown="\"DataType\"" w298 {
              tunnel: w297 -> [w306 w310 w314 w318 w322 w328 w332 w336 w340 w342 w358 w380 w390 w402 w414 w420 w423 w428 w433]
              tunnel: [w306 w309 w313 w317 w321 w327 w331 w335 w339 w347 w360 w379 w389 w401 w413 w419 w425 w427 w432] -> w296
              tunnel: w295 -> [_ w308 w312 w316 w320 w325 w329 w333 w337 w346 w356 w375 w391 w403 w412 w418 w422 w426 w431]
              tunnel: w294 -> [w305 w307 w311 w315 w319 w326 w330 w334 w338 w344 w359 w378 w393 w405 w415 w421 w424 w429 w434]
              tunnel: [w305 w307 w311 w315 w319 w326 w330 w334 w338 w343 w359 w377 w393 w405 w415 w421 w424 w429 w434] -> w293
              frame Default {
              }
              frame "Code" {
                n84 = Bundle By Name(cluster=w310, "Code"=w308) -> (w309:T7)
              }
              frame "Name" {
                n85 = Bundle By Name(cluster=w314, "Name"=w312) -> (w313:T7)
              }
              frame "Description" {
                n86 = Bundle By Name(cluster=w318, "Description"=w316) -> (w317:T7)
              }
              frame "Group" {
                n87 = Bundle By Name(cluster=w322, "Group"=w320) -> (w321:T7)
              }
              frame "IsGroup" {
                n88 = Equal?(x="Yes", y=w325) -> (x = y?=w323:bool)
                n89 = Bundle By Name(cluster=w328, "IsGroup"=w323) -> (w327:T7)
              }
              frame "Tag" {
                n90 = Bundle By Name(cluster=w332, "Tag"=w329) -> (w331:T7)
              }
              frame "Method" {
                n91 = Bundle By Name(cluster=w336, "Method"=w333) -> (w335:T7)
              }
              frame "Parameter" {
                n92 = Bundle By Name(cluster=w340, "Parrameter"=w337) -> (w339:T7)
              }
              frame "DataType" {
                n93 = Unbundle By Name(w342) -> ("IsGroup"=w341:bool)
                n94 = case shown="False" w341 {
                  tunnel: w346 -> [w352 _]
                  tunnel: [w351 DataType."NA" ("DataType")] -> w345
                  tunnel: w344 -> [w350 w354]
                  tunnel: [w349 w354] -> w343
                  frame False {
                    n95 = Scan From String(input string=w352, error in=w350, default 1=DataType."NA" ("DataType")) -> (error out=w349:errorcluster, output 1=w351:T6)  [unwired: 2 in, 2 out]
                  }
                  frame True {
                  }
                }
                n96 = Bundle By Name(cluster=w342, "DataType"=w345) -> (w347:T7)
              }
              frame "Value" {
                n97 = Unbundle By Name(w358) -> ("DataType"=w357:T6)
                n98 = case shown="\"Dbl\"" w357 {
                  tunnel: w356 -> [w362 w366 w370 w372]
                  tunnel: [w361 w363 w367 w373] -> w355
                  frame "String", Default {
                    n99 = To Variant(anything=w362) -> (Variant=w361:variant)
                  }
                  frame "Boolean" {
                    n100 = Equal?(x="1", y=w366) -> (x = y?=w364:bool)
                    n101 = To Variant(anything=w364) -> (Variant=w363:variant)
                  }
                  frame "Int" {
                    n102 = Decimal String To Number(string=w370, default (0L)=i64 0 ("default (0 I32)")) -> (number=w368:i64)  [unwired: 1 in, 1 out]
                    n103 = To Variant(anything=w368) -> (Variant=w367:variant)
                  }
                  frame "Dbl" {
                    n104 = Fract/Exp String To Number(string=w372) -> (number=w371:dbl)  [unwired: 3 in, 1 out]
                    n105 = To Variant(anything=w371) -> (Variant=w373:variant)
                  }
                }
                n106 = Bundle By Name(cluster=w358, "Value"=w355) -> (w360:T7)
              }
              frame "Status" {
                n107 = Empty String/Path?(string/path=w375) -> (empty?=w374:bool)
                n108 = case shown="False" w374 {
                  tunnel: w378 -> [w385 w387]
                  tunnel: [w384 w387] -> w377
                  tunnel: [w382 Status."Pending" ("Status")] -> w376
                  tunnel: w375 -> [w381 _]
                  frame False {
                    n109 = Scan From String(input string=w381, error in=w385, default 1=Status."Pending" ("Status")) -> (error out=w384:errorcluster, output 1=w382:T3)  [unwired: 2 in, 2 out]
                  }
                  frame True {
                  }
                }
                n110 = Bundle By Name(cluster=w380, "Status"=w376) -> (w379:T7)
              }
              frame "LimitLo" {
                n111 = Unbundle By Name(w390) -> ("DataType"=w392:T6)
                n112 = case shown="Default" w392 {
                  tunnel: w391 -> [_ w396 w399]
                  tunnel: [_ w394 w397] -> w388
                  frame Default {
                  }
                  frame "Dbl" {
                    n113 = Fract/Exp String To Number(string=w396) -> (number=w395:dbl)  [unwired: 3 in, 1 out]
                    n114 = To Variant(anything=w395) -> (Variant=w394:variant)
                  }
                  frame "Int" {
                    n115 = Decimal String To Number(string=w399) -> (number=w398:i32)  [unwired: 2 in, 1 out]
                    n116 = To Variant(anything=w398) -> (Variant=w397:variant)
                  }
                }
                n117 = Bundle By Name(cluster=w390, "LimitLo"=w388) -> (w389:T7)
              }
              frame "LimitHi" {
                n118 = Unbundle By Name(w402) -> ("DataType"=w404:T6)
                n119 = case shown="Default" w404 {
                  tunnel: w403 -> [_ w408 w411]
                  tunnel: [_ w406 w409] -> w400
                  frame Default {
                  }
                  frame "Dbl" {
                    n120 = Fract/Exp String To Number(string=w408) -> (number=w407:dbl)  [unwired: 3 in, 1 out]
                    n121 = To Variant(anything=w407) -> (Variant=w406:variant)
                  }
                  frame "Int" {
                    n122 = Decimal String To Number(string=w411) -> (number=w410:i32)  [unwired: 2 in, 1 out]
                    n123 = To Variant(anything=w410) -> (Variant=w409:variant)
                  }
                }
                n124 = Bundle By Name(cluster=w402, "LimitHi"=w400) -> (w401:T7)
              }
              frame "StringMatch" {
                n125 = Bundle By Name(cluster=w414, "StringMatch"=w412) -> (w413:T7)
              }
              frame "BooleanMatch" {
                n126 = Equal?(x="1", y=w418) -> (x = y?=w416:bool)
                n127 = Bundle By Name(cluster=w420, "BooleanMatch"=w416) -> (w419:T7)
              }
              frame "DisplayFormat" {
                n128 = Bundle By Name(cluster=w423, "DisplayFormat"=w422) -> (w425:T7)
              }
              frame "Units" {
                n129 = Bundle By Name(cluster=w428, "Units"=w426) -> (w427:T7)
              }
              frame "TestTime" {
                n130 = Fract/Exp String To Number(string=w431) -> (number=w430:dbl)  [unwired: 3 in, 1 out]
                n131 = Bundle By Name(cluster=w433, "TestTime"=w430) -> (w432:T7)
              }
            }
            n132 = call-poly <vilib>:"Close.vi"("error in (no error)"=w293, "node"=w299) -> ("error out"=w300:errorcluster)  [unwired: 7 in]
          }
        }
        n133 = Bundle By Name(cluster=w281, "Tests"=w279) -> (w280:T1)
      }
    }
  }
  "error out" <- w4
  "Spec" <- w2
